vi "AlliGator Abort.vi"() -> ()   [LabVIEW 2021, in "AlliGator Globals, Variables & Constants.lvlib"]
doc: "Used to interrupt tasks in scripts."
uses:
  AlliGator Globals, Variables & Constants.lvlib
panel:
  out "Abort?":bool
  # "see the AlliGator License on the block diagram (Ctrl+E or Window:Show Block Diagram)"
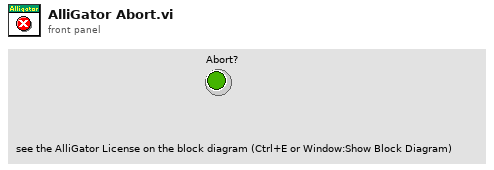
[diagram p1: front panel]
diagram:
